vi "EnterFinish.vi"(10 "Display result?":bool, 11 "Enter finished?":bool) -> (3 "String":string)   [LabVIEW 2020]
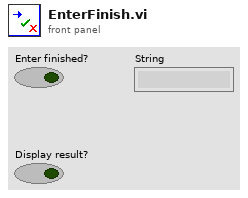
[diagram p1: front panel]
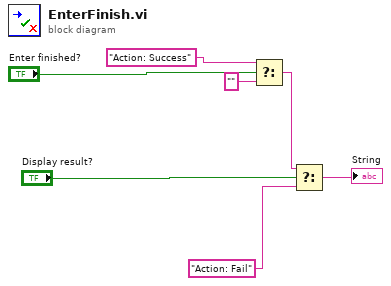
[diagram p0: block diagram]
diagram:
  n1 = Select(t="Action: Success", s="Enter finished?", f="") -> (s? t:f=w3:string)
  n2 = Select(t=w3, s="Display result?", f="Action: Fail") -> (s? t:f=→"String":string)
